vi "open and initialize engine.vi"(6 "timeout in ms":i32=10000, 8 "error in":errorcluster, 10 "engine configuration in":T1, 11 "Target Runtime in":refnum<class "PL_Target Runtime.lvclass">) -> (0 "error out":errorcluster, 2 "Engine Runtime Interface out":refnum<class "Engine Runtime Interface.lvclass">, 3 "Target Runtime out":refnum<class "PL_Target Runtime.lvclass">)   [LabVIEW 2013, in "PL_Target Runtime.lvclass"]
doc: "A helper function which performs the common tasks of loading runtime objects for the engines and modules, and then loading the engine and providing it with associated configuration."
uses:
  PL_Target Runtime.lvclass
  platypus configuration/engines cluster.ctl
  <vilib>/NI/Module Execution Interface/Engine Configuration/engine configuration.lvclass
  <vilib>/NI/Tag Bus Module Framework/module configuration/TBM module configuration.lvclass
  <vilib>/NI/Module Execution Interface/Engine Runtime/Engine Runtime Interface.lvclass
  platypus configuration/PLConfigurationSerializer.lvlib
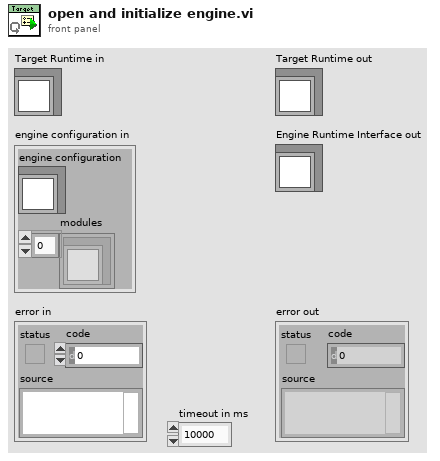
[diagram p1: front panel]
types:
  T1 = typedef "PLConfigurationSerializer.lvlib/engines cluster.ctl" = cluster{"engine configuration":refnum<class "engine configuration.lvclass">, "modules":refnum<class "TBM module configuration.lvclass">[]}
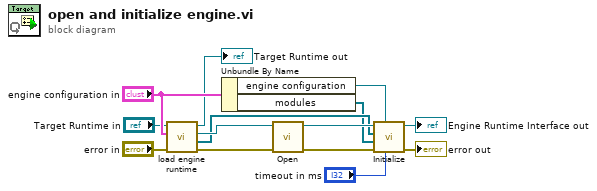
[diagram p0: block diagram]
diagram:
  n1 = call "load engine runtime.vi"("error in"="error in", "engine configuration in"="engine configuration in", "Target Runtime in"="Target Runtime in") -> ("error out"=w11:errorcluster, "Module Runtime Objects"=w10:refnum<class "TBM module execution interface.lvclass">[], "Engine Runtime Object"=w12:refnum<class "Engine Runtime Interface.lvclass">, "Target Runtime out"=→"Target Runtime out":refnum<class "PL_Target Runtime.lvclass">)  [unwired: 5 in]
  n2 = Unbundle By Name("engine configuration in") -> ("engine configuration"=w9:refnum<class "engine configuration.lvclass">, "modules"=w8:refnum<class "TBM module configuration.lvclass">[])
  n3 = call-dynamic "Open.vi"("error in"=w11, "Engine Runtime Interface in"=w12) -> ("error out"=w13:errorcluster, "Engine Runtime Interface out"=w14:refnum<class "Engine Runtime Interface.lvclass">)  [unwired: 8 in]
  n4 = call-dynamic "Initialize.vi"("timeout in ms"="timeout in ms", "Engine Configuration"=w9, "error in"=w13, "module Configurations"=w8, "modules"=w10, "Engine Runtime Interface in"=w14) -> ("error out"=→"error out":errorcluster, "Engine Runtime Interface out"=→"Engine Runtime Interface out":refnum<class "Engine Runtime Interface.lvclass">)  [unwired: 4 in]
